vi "SM Practice.vi"() -> ()   [LabVIEW 2020]
panel:
  out "Numeric":dbl
  in  "stop":bool
  in  "Generate":bool
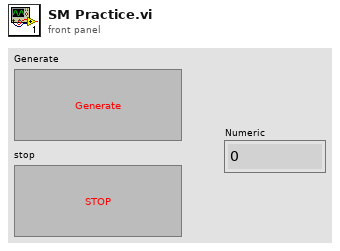
[diagram p1: front panel]
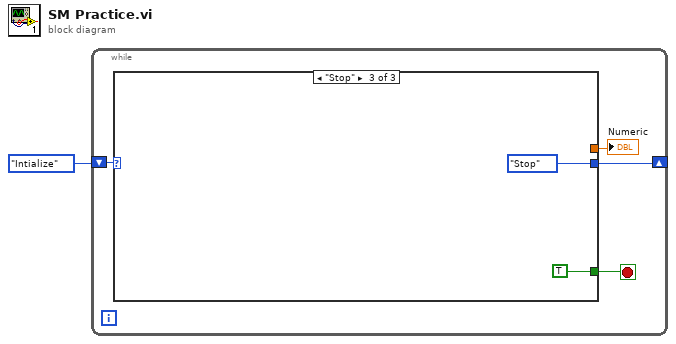
[diagram p0: block diagram]
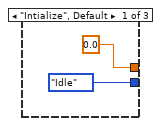
[diagram p2: hidden frame]
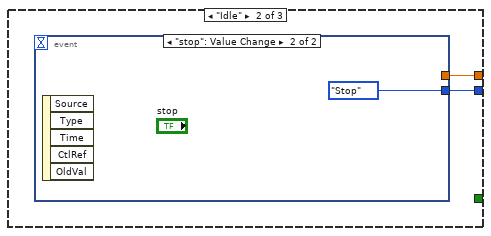
[diagram p3: hidden frame]
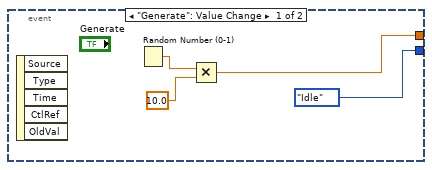
[diagram p4: hidden frame]
diagram:
  n1 = while {
    shift-right: [w4] -> _
    shift-left: enum16{"Intialize", "Idle", "Stop"}."Intialize" -> [w5]
    stop <- w2 stop-if-true
    n2 = case shown="\"Stop\"" w5 {
      tunnel: [enum16{"Intialize", "Idle", "Stop"}."Idle" w8 enum16{"Intialize", "Idle", "Stop"}."Stop"] -> w4
      tunnel: [0.0 w9 _] -> w3
      tunnel: [_ _ TRUE] -> w2
      frame "Intialize", Default {
      }
      frame "Idle" {
        n3 = event shown="[1] \"stop\": Value Change" {
          selector: _ -> [_ _]
          dyn-events: _ -> [_ _]
          timeout: _ -> [_ _]
          tunnel: [w11 _] -> w9
          tunnel: [enum16{"Intialize", "Idle", "Stop"}."Idle" enum16{"Intialize", "Idle", "Stop"}."Stop"] -> w8
          event "Generate": Value Change {
            n4 = event-data() -> ()  [unwired: 1 in, 5 out]
            n5 = Random Number (0-1)() -> (number: 0 to 1=w13:dbl)
            n6 = Multiply(x=w13, y=10.0) -> (x*y=w11:dbl)
          }
          event "stop": Value Change {
            n7 = event-data() -> ()  [unwired: 1 in, 5 out]
          }
        }
      }
      frame "Stop" {
      }
    }
    "Numeric" <- w3
  }
